vi "Control Arm Down.vi"(11 "Avoid Race Condition":bool) -> ()   [LabVIEW 2020]
uses:
  Framework/Robot Global Data.vi
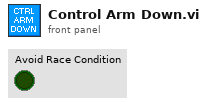
[diagram p1: front panel]
types:
  T1 = typedef "Command Status Info.ctl" = cluster{"Name":string, "Status":T2, "notifier out":T3}
  T2 = typedef "Completion Status.ctl" = enum16{"Successful", "Aborted", "Incomplete"}
  T3 = typedef "Completion Notifier.ctl" = refnum<notifier>
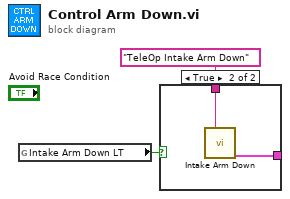
[diagram p0: block diagram]
diagram:
  n1 = global read "Robot Global Data.vi" "Intake Arm Down LT"() -> (w1:bool)
  n2 = case shown="True" w1 {
    tunnel: "TeleOp Intake Arm Down" ("Description") -> [_ w4]
    tunnel: [_ w3] -> _
    frame False {
    }
    frame True {
      n3 = call "Intake Arm Down.vi"("Description"=w4) -> ("Command Info Out"=w3:T1)  [unwired: 10 in]
    }
  }
